vi "Ball Speed Graph Accumulator.vi"(7 "Start Test":bool) -> (0 "cor_pos":sgl format="%.3f", 1 "Vball":dbl format="%.3f", 2 "lat_ball_motion":dbl, 3 "for_ball_motion":dbl, 5 "Total Test Time":dbl=4.01791524887085 format="%.2f", 6 "Chart Ball Speed":cluster{dbl[], dbl[]}[](array[cluster]))   [LabVIEW 2018]
panel:
  out "Chart Ball Speed 2":cluster{dbl[], dbl[]}[](graph) caption="Ball Speed (Vball)"
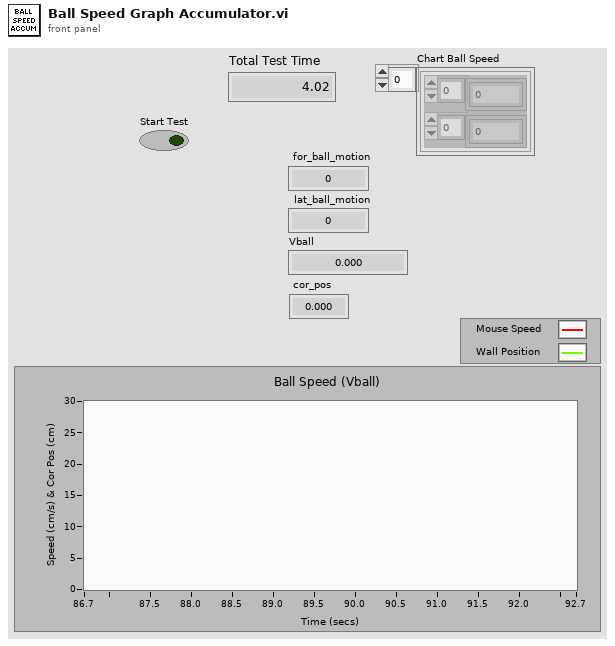
[diagram p1: front panel]
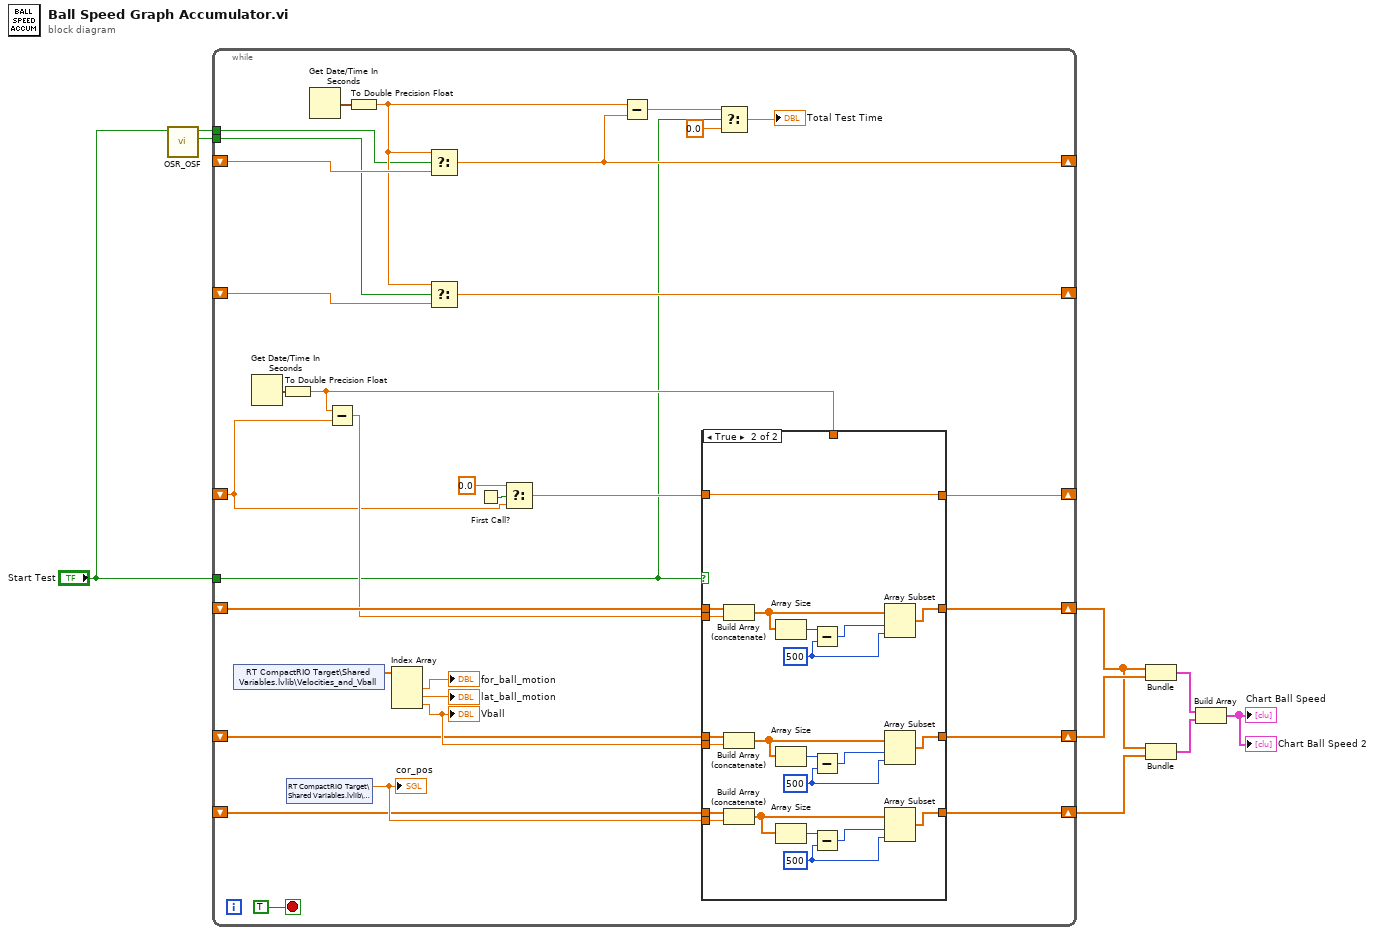
[diagram p0: block diagram]
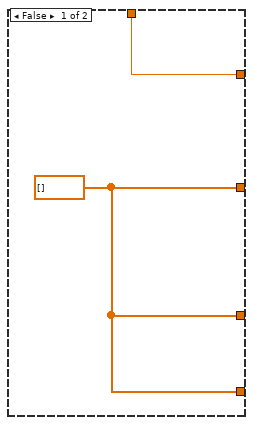
[diagram p2: hidden frame]
diagram:
  n1 = call "OSR_OSF.vi"("BOOL"="Start Test") -> ("OSF"=w2:bool, "OSR"=w3:bool)  [unwired: 9 in]
  n2 = while {
    shift-right: [w11] -> w8
    shift-left: _ -> [w40]
    tunnel: "Start Test" -> [w15]
    shift-right: [w34] -> w9
    shift-left: _ -> [w35]
    shift-right: [w31] -> w7
    shift-left: _ -> [w32]
    shift-right: [w30] -> _
    shift-left: _ -> [w25]
    shift-right: [w16] -> _
    shift-left: _ -> [w21]
    tunnel: w3 -> [w10]
    tunnel: w2 -> [w20]
    shift-right: [w18] -> _
    shift-left: _ -> [w19]
    stop <- TRUE stop-if-true
    n3 = shared-variable "RT CompactRIO Target\\Shared Variables.lvlib\\Velocities_and_Vball"() -> (w39:dbl[])  [unwired: 1 in, 1 out]
    n4 = Get Date/Time In Seconds() -> (seconds since 1Jan1904=w29:timestamp)
    n5 = To Double Precision Float(number=w29) -> (double precision float=w28:dbl)
    n6 = shared-variable "RT CompactRIO Target\\Shared Variables.lvlib\\cor_pos"() -> (w33:sgl)  [unwired: 1 in, 1 out]
    "cor_pos" <- w33
    n7 = Get Date/Time In Seconds() -> (seconds since 1Jan1904=w22:timestamp)
    n8 = Subtract(x=w28, y=w25) -> (x-y=w27:dbl)
    n9 = To Double Precision Float(number=w22) -> (double precision float=w17:dbl)
    n10 = Index Array(array=w39) -> (element #1=→"for_ball_motion":dbl, element #2=→"lat_ball_motion":dbl, element #3=w36:dbl)  [unwired: 3 in]
    "Vball" <- w36
    n11 = Select(t=w17, s=w10, f=w21) -> (s? t:f=w16:dbl)
    n12 = Select(t=w17, s=w20, f=w19) -> (s? t:f=w18:dbl)
    n13 = First Call?() -> (First Call?: T/F=w26:bool)
    n14 = Select(t=0.0, s=w26, f=w25) -> (s? t:f=w24:dbl)
    n15 = Subtract(x=w17, y=w16) -> (x-y=w14:dbl)
    n16 = case shown="True" w15 {
      tunnel: w27 -> [_ w64]
      tunnel: w40 -> [_ w65]
      tunnel: [w43 w58] -> w11
      tunnel: w36 -> [_ w63]
      tunnel: w35 -> [_ w62]
      tunnel: [w43 w47] -> w34
      tunnel: w33 -> [_ w61]
      tunnel: w32 -> [_ w60]
      tunnel: [w43 w44] -> w31
      tunnel: [w42 w59] -> w30
      tunnel: w24 -> [_ w59]
      tunnel: w28 -> [w42 _]
      frame False {
        w43 = dbl[] []
      }
      frame True {
        w48 = 500 ("length")
        w53 = 500 ("length")
        w54 = 500 ("length")
        n17 = Build Array (concatenate)(w65, w64) -> (w56:dbl[])
        n18 = Build Array (concatenate)(w62, w63) -> (w45:dbl[])
        n19 = Build Array (concatenate)(w60, w61) -> (w46:dbl[])
        n20 = Array Size(array=w56) -> (size(s)=w57:i32)
        n21 = Array Size(array=w45) -> (size(s)=w51:i32)
        n22 = Array Size(array=w46) -> (size(s)=w50:i32)
        n23 = Subtract(x=w57, y=w54) -> (x-y=w55:i32)
        n24 = Subtract(x=w51, y=w53) -> (x-y=w52:i32)
        n25 = Subtract(x=w50, y=w48) -> (x-y=w49:i32)
        n26 = Array Subset(array=w56, index=w55, length=w54) -> (w58:dbl[])
        n27 = Array Subset(array=w45, index=w52, length=w53) -> (w47:dbl[])
        n28 = Array Subset(array=w46, index=w49, length=w48) -> (w44:dbl[])
      }
    }
    n29 = Select(t=w14, s=w15, f=0.0) -> (s? t:f=→"Total Test Time":dbl)
  }
  n30 = Bundle(w8, w9) -> (w6:cluster{dbl[], dbl[]})  [unwired: 1 in]
  n31 = Bundle(w8, w7) -> (w5:cluster{dbl[], dbl[]})  [unwired: 1 in]
  n32 = Build Array(w6, w5) -> (→"Chart Ball Speed" →"Chart Ball Speed 2":cluster{dbl[], dbl[]}[])
